vi "edittest format sequence form to record.vi"(6 "User":T1, 8 "error in (no error)":errorcluster, 9 "Sequence POST (empty)":T7, 10 "Sequence Record In":T2, 11 "Connection Refnum":T3) -> (0 "error out":errorcluster, 1 "Sequence Fields":T4[](array[typedef]), 2 "Sequence Record":T2, 3 "dup Connection Refnum":T3, 5 "sxSequenceId Delete":string)   [LabVIEW 2011]
uses:
  Addons/internet/utils/keyedarr.llb/Keyed Array.ctl
  server/database/Sequences/Sequence Record.ctl
  server/database/Fields/Field Record.ctl
  server/database/Fields/Field DataTypes.ctl
  server/database/Fields/Field NextItem.ctl
  SI.LIB/ODBC/SQL Controls/Connection Refnum.ctl
  server/database/Users/User Record.ctl
  Addons/internet/utils/strutil.llb/Case Matching.ctl
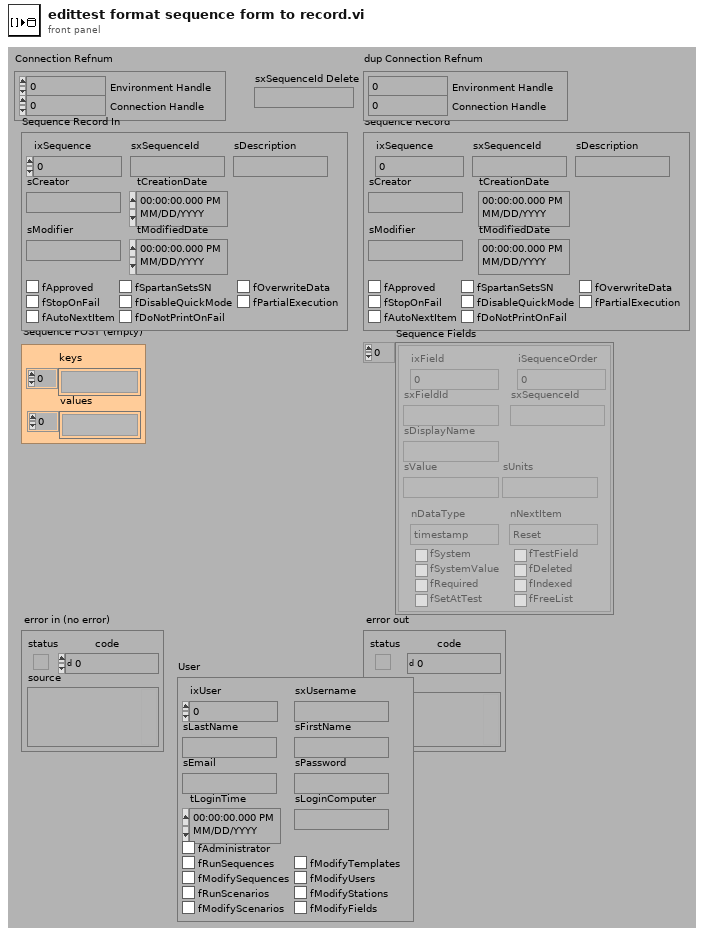
[diagram p1: front panel]
types:
  T1 = typedef "User Record.ctl" = cluster{"ixUser":i32, "sxUsername":string, "sLastName":string, "sFirstName":string, "sEmail":string, "sPassword":string, "tLoginTime":timestamp, "sLoginComputer":string, "fAdministrator":bool, "fRunSequences":bool, "fModifySequences":bool, "fRunScenarios":bool, "fModifyScenarios":bool, "fModifyTemplates":bool, "fModifyUsers":bool, "fModifyStations":bool, "fModifyFields":bool}
  T2 = typedef "Sequence Record.ctl" = cluster{"ixSequence":i32, "sxSequenceId":string, "sDescription":string, "sCreator":string, "tCreationDate":timestamp, "sModifier":string, "tModifiedDate":timestamp, "fApproved":bool, "fSpartanSetsSN":bool, "fOverwriteData":bool, "fStopOnFail":bool, "fDisableQuickMode":bool, "fPartialExecution":bool, "fAutoNextItem":bool, "fDoNotPrintOnFail":bool}
  T3 = typedef "Connection Refnum.ctl" = cluster{"Environment Handle":i32, "Connection Handle":i32}
  T4 = typedef "Field Record.ctl" = cluster{"ixField":i32, "iSequenceOrder":i32, "sxFieldId":string, "sxSequenceId":string, "sDisplayName":string, "sValue":string, "sUnits":string, "nDataType":T5, "nNextItem":T6, "fSystem":bool, "fSystemValue":bool, "fRequired":bool, "fSetAtTest":bool, "fTestField":bool, "fDeleted":bool, "fIndexed":bool, "fFreeList":bool}
  T5 = typedef "Field DataTypes.ctl" = enum32{"text", "numeric", "list", "timestamp", "boolean"}
  T6 = typedef "Field NextItem.ctl" = enum32{"Reset", "Retain", "Auto-Increment"}
  T7 = typedef "Keyed Array.ctl" = cluster{"keys":string[], "values":string[]}
  T8 = typedef "Case Matching.ctl" = enum16{"a != A", "a == A", "system"}
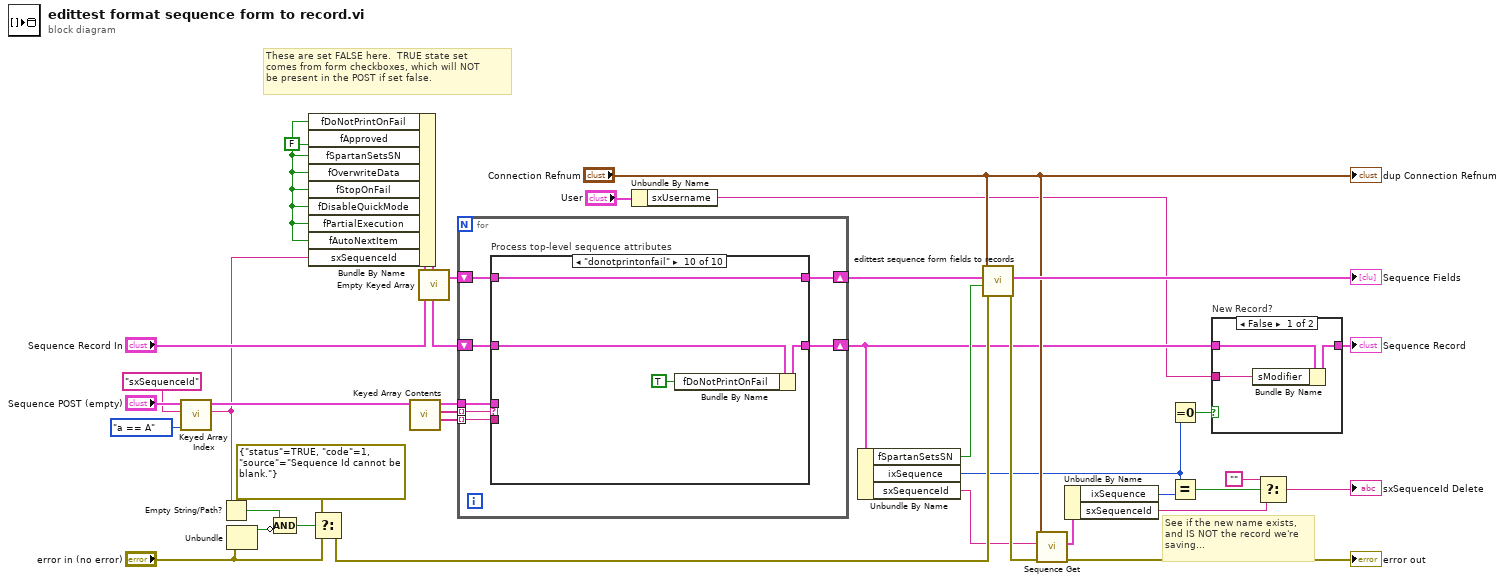
[diagram p0: block diagram]
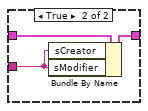
[diagram p2: hidden frame]
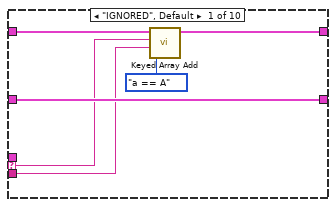
[diagram p3: hidden frame]
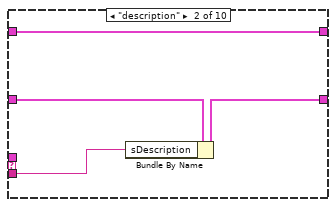
[diagram p4: hidden frame]
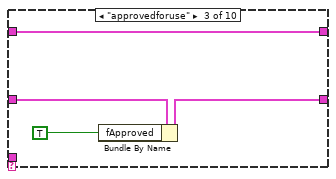
[diagram p5: hidden frame]
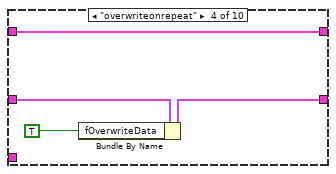
[diagram p6: hidden frame]
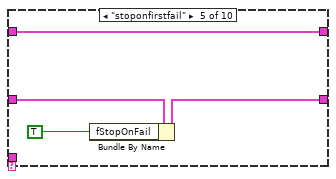
[diagram p7: hidden frame]
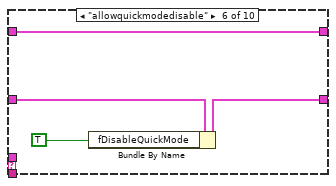
[diagram p8: hidden frame]
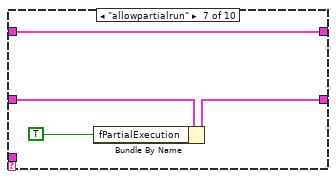
[diagram p9: hidden frame]
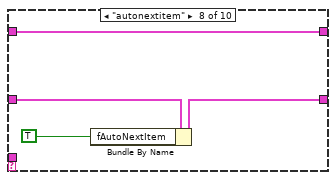
[diagram p10: hidden frame]
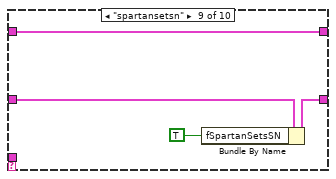
[diagram p11: hidden frame]
diagram:
  w1 = FALSE
  # "See if the new name exists,\nand IS NOT the record we're\nsaving..."
  # "These are set FALSE here.  TRUE state set\ncomes from form checkboxes, which will NOT\nbe present in the POST if set false."
  n1 = call "Keyed Array Index.vi"("case matching (sensitive)"=Case_Matching."a == A", "key"="sxSequenceId", "array in"="Sequence POST (empty)") -> ("value"=w18:string, "duplicate array"=w27:T7)  [unwired: 1 in, 2 out]
  n2 = Empty String/Path?(string/path=w18) -> (empty?=w24:bool)
  n3 = Unbundle("error in (no error)") -> ("status"=w23:bool)  [unwired: 2 out]
  n4 = Compound Arithmetic op=AND(w24, invert w23) -> (w22:bool)
  n5 = Bundle By Name(cluster="Sequence Record In", "fDoNotPrintOnFail"=w1, "fApproved"=w1, "fSpartanSetsSN"=w1, "fOverwriteData"=w1, "fStopOnFail"=w1, "fDisableQuickMode"=w1, "fPartialExecution"=w1, "fAutoNextItem"=w1, "sxSequenceId"=w18) -> (w29:T2)
  n6 = Select(t=errorcluster {"status"=TRUE, "code"=1, "source"="Sequence Id cannot be blank."}, s=w22, f="error in (no error)") -> (s? t:f=w20:errorcluster)
  n7 = call "Keyed Array Contents.vi"("array in"=w27) -> ("values"=w36:string[], "keys"=w37:string[], "duplicate array"=w35:T7)  [unwired: 4 out]
  n8 = call "Empty Keyed Array.vi"() -> ("empty keyed array"=w34:T7)  [unwired: 3 out]
  n9 = for {
    tunnel: w37 -> [w41] mode=indexing
    tunnel: w36 -> [w40] mode=indexing
    shift-right: [w43] -> w9
    shift-left: w29 -> [w44]
    tunnel: w35 -> [w42]
    shift-right: [w38] -> w33
    shift-left: w34 -> [w39]
    n10 = case "Process top-level sequence attributes" shown="\"donotprintonfail\"" w41 {
      selector: w41 -> [w48 _ _ _ _ _ _ _ _ _]
      tunnel: w44 -> [w50 w54 w58 w62 w66 w70 w74 w78 w81 w85]
      tunnel: [w50 w53 w57 w61 w65 w69 w73 w77 w82 w86] -> w43
      tunnel: w42 -> [_ _ _ _ _ _ _ _ _ _]
      tunnel: w40 -> [w47 w52 _ _ _ _ _ _ _ _]
      tunnel: w39 -> [w49 w51 w55 w59 w63 w67 w71 w75 w80 w84]
      tunnel: [w45 w51 w55 w59 w63 w67 w71 w75 w80 w84] -> w38
      frame "IGNORED", Default {
        n11 = call "Keyed Array Add.vi"("case matching (sensitive)"=Case_Matching."a == A", "value"=w47, "key"=w48, "array in"=w49) -> ("array out"=w45:T7)  [unwired: 3 out]
      }
      frame "description" {
        n12 = Bundle By Name(cluster=w54, "sDescription"=w52) -> (w53:T2)
      }
      frame "approvedforuse" {
        n13 = Bundle By Name(cluster=w58, "fApproved"=TRUE) -> (w57:T2)
      }
      frame "overwriteonrepeat" {
        n14 = Bundle By Name(cluster=w62, "fOverwriteData"=TRUE) -> (w61:T2)
      }
      frame "stoponfirstfail" {
        n15 = Bundle By Name(cluster=w66, "fStopOnFail"=TRUE) -> (w65:T2)
      }
      frame "allowquickmodedisable" {
        n16 = Bundle By Name(cluster=w70, "fDisableQuickMode"=TRUE) -> (w69:T2)
      }
      frame "allowpartialrun" {
        n17 = Bundle By Name(cluster=w74, "fPartialExecution"=TRUE) -> (w73:T2)
      }
      frame "autonextitem" {
        n18 = Bundle By Name(cluster=w78, "fAutoNextItem"=TRUE) -> (w77:T2)
      }
      frame "spartansetsn" {
        n19 = Bundle By Name(cluster=w81, "fSpartanSetsSN"=TRUE) -> (w82:T2)
      }
      frame "donotprintonfail" {
        n20 = Bundle By Name(cluster=w85, "fDoNotPrintOnFail"=TRUE ("fSpartanSetsSN")) -> (w86:T2)
      }
    }
  }
  n21 = Unbundle By Name("User") -> ("sxUsername"=w7:string)
  n22 = Unbundle By Name(w9) -> ("fSpartanSetsSN"=w31:bool, "ixSequence"=w11:i32, "sxSequenceId"=w15:string)
  n23 = call "edittest sequence form fields to records.vi"("error in (no error)"=w20, "fSpartanSetsSN"=w31, "Sequence FIELDs POST (empty)"=w33, "Connection Refnum"="Connection Refnum") -> ("error out"=w16:errorcluster, "Sequence Fields"=→"Sequence Fields":T4[])  [unwired: 6 out]
  n24 = call "Sequence Get.vi"("error in (no error)"=w16, "sxSequenceId (\"\")"=w15, "Connection Refnum"="Connection Refnum") -> ("error out"=→"error out":errorcluster, "Sequence Record"=w13:T2)  [unwired: 7 out]
  n25 = Unbundle By Name(w13) -> ("ixSequence"=w17:i32, "sxSequenceId"=w4:string)
  n26 = Equal To 0?(x=w11) -> (x = 0?=w10:bool)
  n27 = Equal?(x=w11, y=w17) -> (x = y?=w5:bool)
  n28 = case "New Record?" shown="False" w10 {
    tunnel: w9 -> [w89 w92]
    tunnel: [w88 w91] -> w8
    tunnel: w7 -> [w87 w90]
    frame False {
      n29 = Bundle By Name(cluster=w89, "sModifier"=w87) -> (w88:T2)
    }
    frame True {
      n30 = Bundle By Name(cluster=w92, "sCreator"=w90, "sModifier"=w90) -> (w91:T2)
    }
  }
  "Sequence Record" <- w8
  n31 = Select(t="", s=w5, f=w4) -> (s? t:f=→"sxSequenceId Delete":string)
  "dup Connection Refnum" <- "Connection Refnum"
